vi "FTW-Socket-Core-LibraryFilepath.vi"(8 "error in":errorcluster) -> (0 "error out":errorcluster, 1 "Library Version":string, 2 "Library Filepath":path)   [LabVIEW 2013]
uses:
  error/FTW-ERR-ThrowError.vi
  error/FTW-ERR-NoErrorConstant.vi
  error/FTW-ERR-CallChain.vi
  string/FTW-STR-ReplaceWhitespace.vi
  lib/nanomsg/FTWLib-nanomsg-Win32.vi
  lib/nanomsg/FTWLib-nanomsg-LinuxRT.vi
  lib/nanomsg/FTWLib-nanomsg-Win64.vi
panel:
  # "Inputs"
  # "Outputs"
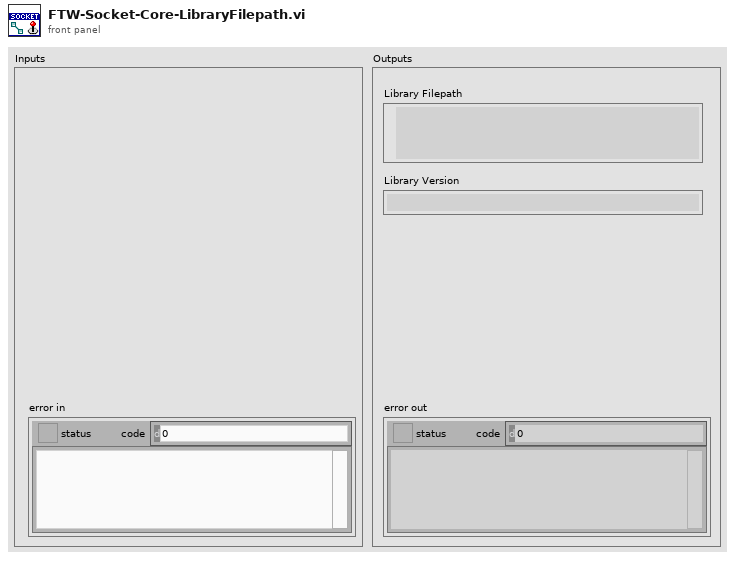
[diagram p1: front panel]
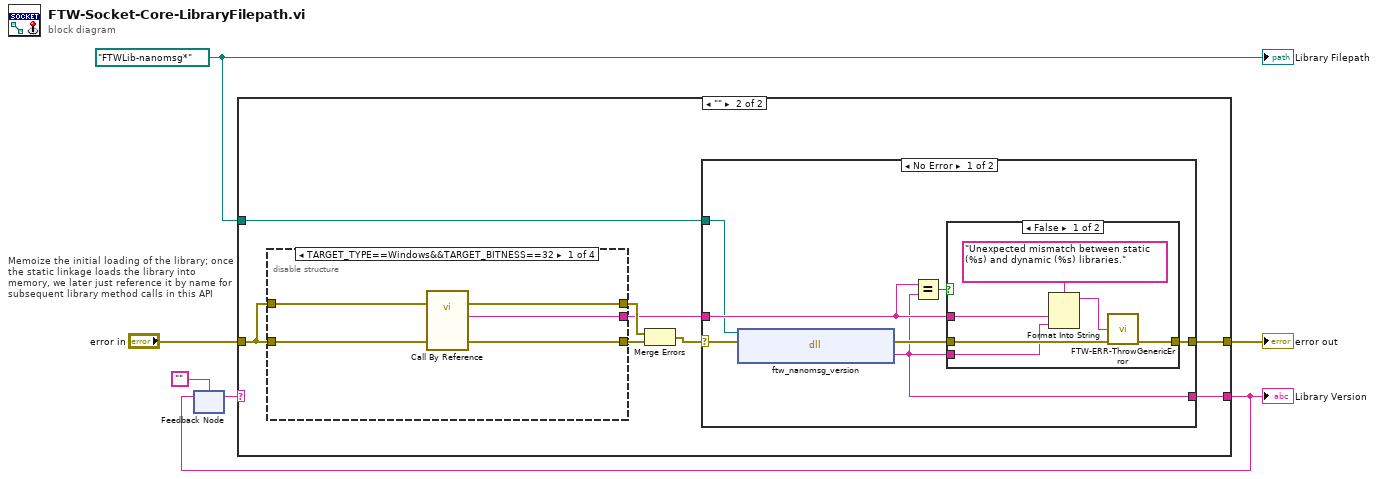
[diagram p0: block diagram]
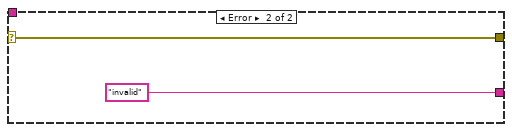
[diagram p4: hidden frame]
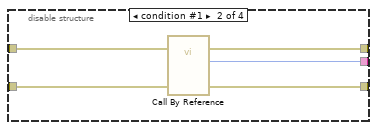
[diagram p5: hidden frame]
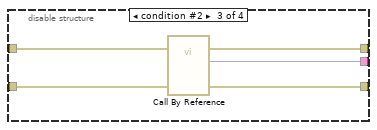
[diagram p6: hidden frame]
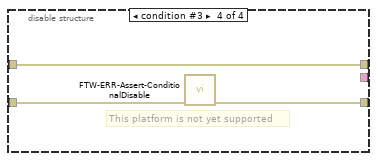
[diagram p7: hidden frame]
diagram:
  w1 = path "FTWLib-nanomsg*" ("nanomsg Library Filepath")
  n1 = feedback #1("") -> (w3:string)
  n2 = case "Memoize the initial loading of the library; once the static linkage loads the library into memory, we later just reference it by name for subsequent library method calls in this API" shown="\"\"" w3 {
    selector: w3 -> [w7 _]
    tunnel: "error in" -> [w8 w12]
    tunnel: [w7 w15] -> w4
    tunnel: [w8 w16] -> w5
    tunnel: w1 -> [_ w10]
    frame Default {
    }
    frame "" {
      n3 = disable-structure shown="TARGET_TYPE==Windows&&TARGET_BITNESS==32" {
        disable-tunnel: [w37 w39 w44 _] -> w9
        disable-tunnel: [w36 w38 w43 w49] -> w13
        disable-tunnel: w12 -> [w34 w41 w46 w50]
        disable-tunnel: [w35 w40 w45 w48] -> w14
        disable-tunnel: w12 -> [w33 w42 w47 w48]
        frame condition #0 (active) {
          n4 = call-by-ref "?"(error in=w33, "error in"=w34) -> (error out=w35:errorcluster, "Library Version"=w37:string, 15:"error out"=w36:errorcluster)  [unwired: 14 in, 1 out]
        }
        frame condition #1 {
          n5 = call-by-ref "?"(error in=w42, "error in"=w41) -> (error out=w40:errorcluster, "Integer Size"=w39:i32, 15:"error out"=w38:errorcluster)  [unwired: 14 in, 1 out]
        }
        frame condition #2 {
          n6 = call-by-ref "?"(error in=w47, "error in"=w46) -> (error out=w45:errorcluster, "Integer Size"=w44:i32, 15:"error out"=w43:errorcluster)  [unwired: 14 in, 1 out]
        }
        frame condition #3 {
          # "This platform is not yet supported"
          n7 = call "FTW-ERR-Assert-ConditionalDisable.vi"("error in"=w50) -> ("error out"=w49:errorcluster)  [unwired: 14 in]
        }
      }
      n8 = Merge Errors(w14, w13) -> (w11:errorcluster)
      n9 = case shown="No Error" w11 {
        selector: w11 -> [w23 w31]
        tunnel: [w20 w31] -> w16
        tunnel: [w18 "invalid" ("Version (minus Build)")] -> w15
        tunnel: w10 -> [w17 _]
        tunnel: w9 -> [w19 _]
        frame No Error {
          n10 = dll-call lib="?" fn="ftw_nanomsg_version"(path in=w17, error in=w23) -> (error out=w21:errorcluster, "FTW-nanomsg Version"=w18:string)  [unwired: 1 in, 1 out]
          n11 = Equal?(x=w19, y=w18) -> (x = y?=w22:bool)
          n12 = case shown="False" w22 {
            tunnel: w21 -> [w29 w30]
            tunnel: [w28 w30] -> w20
            tunnel: w19 -> [w26 _]
            tunnel: w18 -> [w25 _]
            frame False {
              n13 = Format Into String(format string="Unexpected mismatch between static (%s) and dynamic (%s) libraries.", w26, w25) -> (resulting string=w24:string)  [unwired: 2 in, 1 out]
              n14 = call "FTW-ERR-ThrowGenericError.vi"("Error Message"=w24, "error in"=w29) -> ("error out"=w28:errorcluster)  [unwired: 13 in]
            }
            frame True {
            }
          }
        }
        frame Error {
        }
      }
    }
  }
  "error out" <- w5
  "Library Version" <- w4
  n15 = feedback-in #1(w4) -> ()
  "Library Filepath" <- w1
